vi "Led multicolor.vi"() -> ()   [LabVIEW 2024]
panel:
  out "Color Circle Box":u32(colorbox) caption="Color Box"
  out "multicolor box":u32(colorbox)
  out "desconectado":bool
  out "fuera de servicio":bool
  out "mantenimiento":bool
  out "avería":bool
  out "funcionando":bool
  in  "Terminar":bool
  out "Multiled":bool
  out "opciones ind":T1(tab)
  in  "opciones":T1(radio)
  # "Nodo de propiedad"
  # "Tab Control"
  # "Muchos led's"
  # "Color box"
  # "Color box personalizado"
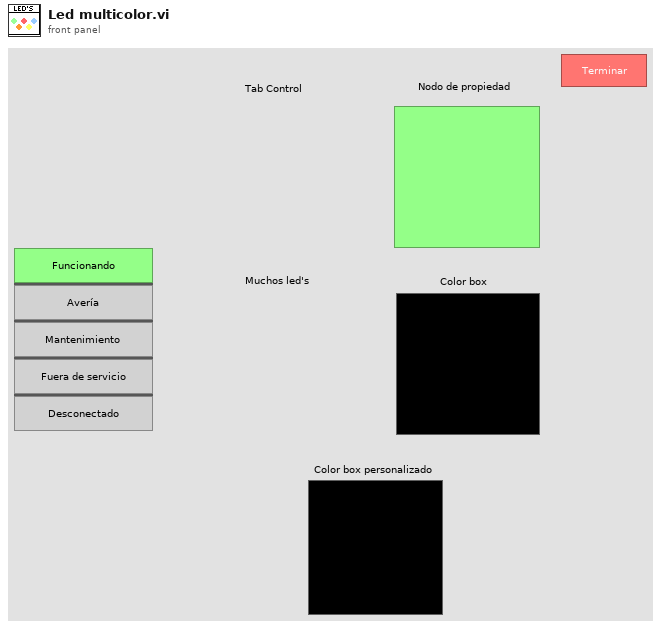
[diagram p1: front panel]
types:
  T1 = enum32{"Funcionando ctl", "avería ctl", "mantenimiento ctl", "fuera de servicio ctl", "desconectado ctl"}
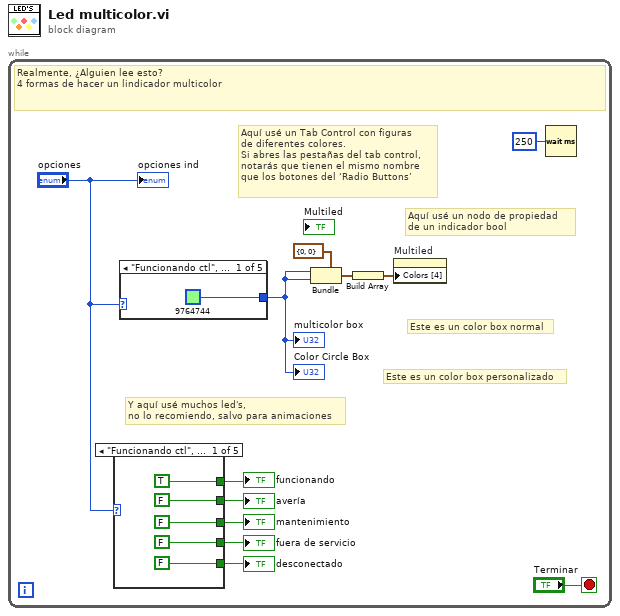
[diagram p0: block diagram]
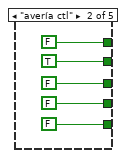
[diagram p2: hidden frame]
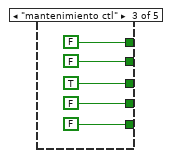
[diagram p3: hidden frame]
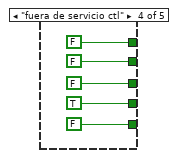
[diagram p4: hidden frame]
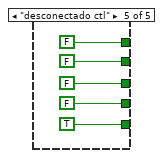
[diagram p5: hidden frame]
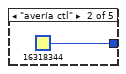
[diagram p6: hidden frame]
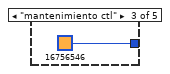
[diagram p7: hidden frame]
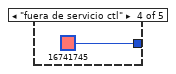
[diagram p8: hidden frame]
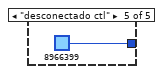
[diagram p9: hidden frame]
diagram:
  n1 = while {
    stop <- "Terminar" stop-if-true
    # "Y aquí usé muchos led's,\nno lo recomiendo, salvo para animaciones"
    # "Este es un color box personalizado"
    # "Este es un color box normal"
    # "Aquí usé un nodo de propiedad\nde un indicador bool"
    # "Aquí usé un Tab Control con figuras\nde diferentes colores.\nSi abres las pestañas del tab control,\nnotarás que tienen el mismo nombre\nque los botones del ‘Radio Buttons’"
    # "Realmente, ¿Alguien lee esto?\n4 formas de hacer un lindicador multicolor"
    n2 = case shown="\"Funcionando ctl\", Default" "opciones" {
      tunnel: [TRUE FALSE FALSE FALSE FALSE] -> w7
      tunnel: [FALSE TRUE FALSE FALSE FALSE] -> w6
      tunnel: [FALSE FALSE TRUE FALSE FALSE] -> w5
      tunnel: [FALSE FALSE FALSE TRUE FALSE] -> w4
      tunnel: [FALSE FALSE FALSE FALSE TRUE] -> w3
      frame "Funcionando ctl", Default {
      }
      frame "avería ctl" {
      }
      frame "mantenimiento ctl" {
      }
      frame "fuera de servicio ctl" {
      }
      frame "desconectado ctl" {
      }
    }
    "funcionando" <- w7
    "mantenimiento" <- w5
    "avería" <- w6
    "fuera de servicio" <- w4
    "desconectado" <- w3
    n3 = case shown="\"Funcionando ctl\", Default" "opciones" {
      tunnel: [u32 9764744 u32 16318344 u32 16756546 u32 16741745 u32 8966399] -> w1
      frame "Funcionando ctl", Default {
      }
      frame "avería ctl" {
      }
      frame "mantenimiento ctl" {
      }
      frame "fuera de servicio ctl" {
      }
      frame "desconectado ctl" {
      }
    }
    "multicolor box" <- w1
    "Color Circle Box" <- w1
    n4 = Bundle(cluster=cluster{i32, i32} {0, 0}, w1, w1) -> (w12:cluster{i32, i32})
    n5 = Build Array(w12) -> (w11:cluster{i32, i32}[])
    n6 = property on="Multiled" class="Bool (strict)"("Colors [4]"=w11) -> ()  [unwired: 2 in, 2 out]
    n7 = Wait (ms)(milliseconds to wait=u32 250) -> ()  [unwired: 1 out]
    "opciones ind" <- "opciones"
  }
